vi "Ready to fire.vi"() -> (3 "READY TO FIRE":bool)   [LabVIEW 2012]
uses:
  Team Code/Robot Global Data.vi
panel:
  in  "stop":bool
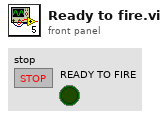
[diagram p1: front panel]
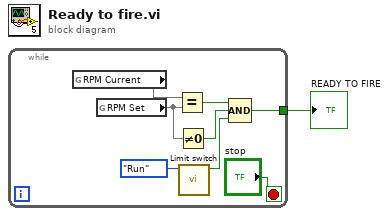
[diagram p0: block diagram]
diagram:
  n1 = while {
    tunnel: [w5] -> w1
    stop <- "stop" stop-if-true
    n2 = global read "Robot Global Data.vi" "RPM Current"() -> (w3)
    n3 = global read "Robot Global Data.vi" "RPM Set"() -> (w2)
    n4 = Equal?(x=w3, y=w2) -> (x = y?=w8:bool)
    n5 = Not Equal To 0?(x=w2) -> (x != 0?=w7:bool)
    n6 = call "Limit switch.vi"("Enum"=enum16{"Start", "Run", "End"}."Run") -> ("Value"=w6:bool)  [unwired: 10 in]
    n7 = Compound Arithmetic op=AND(w8, w7, w6) -> (w5:bool)
  }
  "READY TO FIRE" <- w1
